vi "Add Parameter.vi"(8 "error in (no error)":errorcluster, 9 "Type (Output)":T1=enum."Output", 10 "parameter":T3 {"Parameter"."encoding" items=["BNR", "BCD", "Discrete", "Signed_32", "Signed_64", "Float_32", "Float_64", "Opaque"]}, 11 "section ref in":T2 format="%.0x") -> (0 "error out":errorcluster, 3 "section ref out":T2 format="%.0x")   [LabVIEW 2020, in "AIM ARINC 664 Scripting.lvlib"]
uses:
  AIM ARINC 664 Scripting.lvlib
  <vilib>/NI VeriStand/Custom Device API/Custom Device API.lvlib
  <vilib>/NI VeriStand/Custom Device API/Custom Device Channel Type.ctl
  <vilib>/NI VeriStand/Custom Device API/Custom Device Channel.ctl
  Shared/Encoding (Arinc664).ctl
  Import/_typedefs/frame_parameter_definition.ctl
  Import/AIM ARINC 664 Import.lvlib
  Import/_typedefs/frame_parameter.ctl
  <vilib>/NI VeriStand/Custom Device API/Custom Device Item Ref.ctl
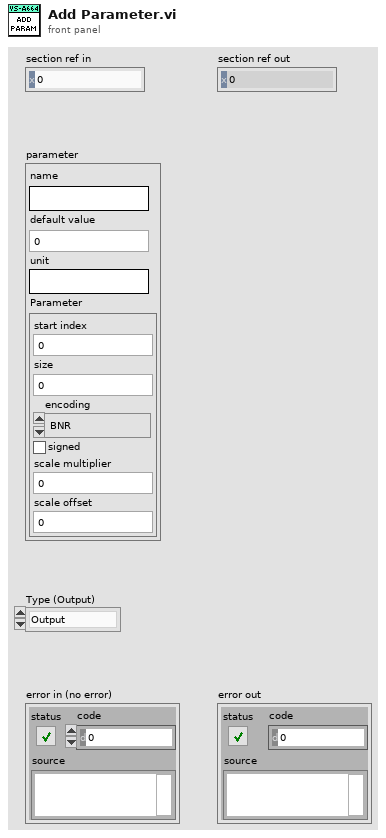
[diagram p1: front panel]
types:
  T1 = typedef "Custom Device API.lvlib/Custom Device Channel Type.ctl" = enum16{"Input", "Output"}
  T2 = typedef "Custom Device API.lvlib/Custom Device Item Ref.ctl" = u64
  T3 = typedef "AIM ARINC 664 Import.lvlib/frame_parameter.ctl" = cluster{"name":string, "default value":dbl, "unit":string, "Parameter":T4}
  T4 = typedef "AIM ARINC 664 Import.lvlib/frame_parameter_definition.ctl" = cluster{"start index":i32, "size":i32, "encoding":T5, "signed":bool, "scale multiplier":dbl, "scale offset":dbl}
  T5 = typedef "Encoding (Arinc664).ctl" = u16
  T6 = typedef "Custom Device API.lvlib/Custom Device Channel.ctl" = cluster{"Type":T1, "Units":string, "Default Value":dbl, "Faultable":bool, "Scalable":bool}
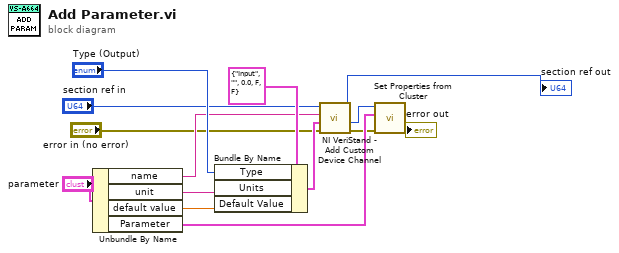
[diagram p0: block diagram]
diagram:
  n1 = Unbundle By Name("parameter") -> ("name"=w5:string, "unit"=w8:string, "default value"=w9:dbl, "Parameter"=w12:T4)
  n2 = Bundle By Name(cluster=T6 {"Type"=enum."Input", "Units"="", "Default Value"=0.0, "Faultable"=FALSE, "Scalable"=FALSE} ("Channel"), "Type"="Type (Output)", "Units"=w8, "Default Value"=w9) -> (w7:T6)
  n3 = call <vilib>:"NI VeriStand - Add Custom Device Channel.vi"("error in (no error)"="error in (no error)", "Channel"=w7, "Channel Name"=w5, "Parent Ref in"="section ref in") -> ("error out"=w10:errorcluster, "Channel Ref"=w13:T2, "Parent Ref out"=→"section ref out":T2)  [unwired: 4 in, 1 out]
  n4 = call "Set Properties from Cluster.vi"("error in"=w10, "Variant Cluster"=w12, "item ref in"=w13) -> ("error out"=→"error out":errorcluster)  [unwired: 7 in, 1 out]
